vi "CAN Jaguar Clear Ack.vi"(8 "DevStatus":errorcluster, 11 "Device Number":u8) -> (0 "error out":errorcluster)   [LabVIEW 2009, in "CAN.lvlib"]
uses:
  CAN.lvlib
  CAN Motor Message IDs.ctl
  Serial.lvlib
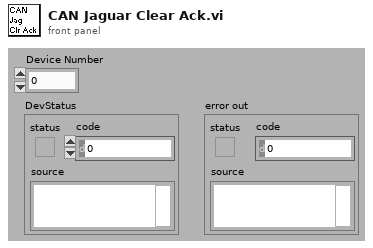
[diagram p1: front panel]
types:
  T1 = typedef "CAN.lvlib/CAN Motor Message IDs.ctl" = u32
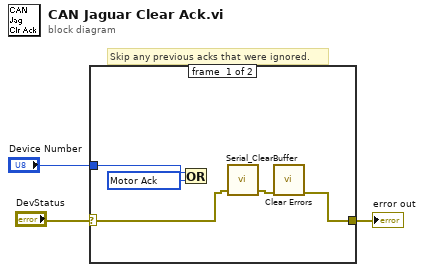
[diagram p0: block diagram]
diagram:
  # "Skip any previous acks that were ignored."
  n1 = case shown="No Error" "DevStatus" {
    selector: "DevStatus" -> [w5 w9]
    tunnel: [w6 w9] -> w3
    tunnel: "Device Number" -> [w8 _]
    frame #0 {
      w7 = T1 33693696 items=["Volt Enable"=33685504, "Volt Disable"=33685568, "Volt Set"=33685632, "Volt Set Ramp"=33685696, "Speed Enable"=33686528, "Speed Disable"=33686592, "Speed Set"=33686656, "Speed P"=33686720, "Speed I"=33686784, "Speed D"=33686848, "Speed Ref"=33686912, "Position Enable"=33688576, "Position Disable"=33688640, "Position Set"=33688704, "Position P"=33688768, "Position I"=33688832, "Position D"=33688896, "Position Ref"=33688960, "Current Enable"=33689600, "Current Disable"=33689664, "Current Set"=33689728, "Current P"=33689792, "Current I"=33689856, "Current D"=33689920, "Status VOut"=33690624, "Status VBus"=33690688, "Status Current"=33690752, "Status Temp"=33690816, "Status Position"=33690880, "Status Speed"=33690944, "Status Limit"=33691008, "Status Fault"=33691072, "Status Power"=33691136, "Config Num Brushes"=33692672, "Config Encoder Lines"=33692736, "Config Pot Turns"=33692800, "Config Brake Coast"=33692864, "Config Limit Mode"=33692928, "Config Limit Fwd"=33692992, "Config Limit Rev"=33693056, "Config Max VOut"=33693120, "Config Fault Time"=33693184, "Motor Ack"=33693696] ("CAN Motor Message IDs")
      n2 = Or(x=w8, y=w7) -> ()  [unwired: 1 out]
      n3 = call "Serial_ClearBuffer.vi"("error in (no error)"=w5) -> ("error out"=w4:errorcluster)  [unwired: 3 in, 1 out]
      n4 = call <vilib>:"Clear Errors.vi"("error in (no error)"=w4) -> ("error out"=w6:errorcluster)  [unwired: 6 out]
    }
    frame #1 {
    }
  }
  "error out" <- w3
